vi "Test Analog Channel.vi"(8 "error in (no error)":errorcluster, 9 "Channel (0)":u32, 10 "Test Label":string, 11 "CT Common Tests in":refnum<class "CT Common Tests.lvclass">) -> (0 "error out":errorcluster, 1 "Result":string, 2 "Passed":bool, 3 "CT Common Tests out":refnum<class "CT Common Tests.lvclass">)   [LabVIEW 2015, in "CT Common Tests.lvclass"]
uses:
  CT Common Tests.lvclass
  Classes/Instruments/MIO Device/MIO Device/Class/typedefs/Read Type -- Enum.ctl
  Classes/Instruments/MIO Device/MIO Device/Class/typedefs/Channel Type -- Enum.ctl
  Classes/Instruments/MIO Device/MIO Device/Class/MIO Device.lvclass
  Classes/Application/Class/Application.lvclass
  Classes/Test Recipe/Class/Test Recipe.lvclass
  Test Class/Test Class.lvclass
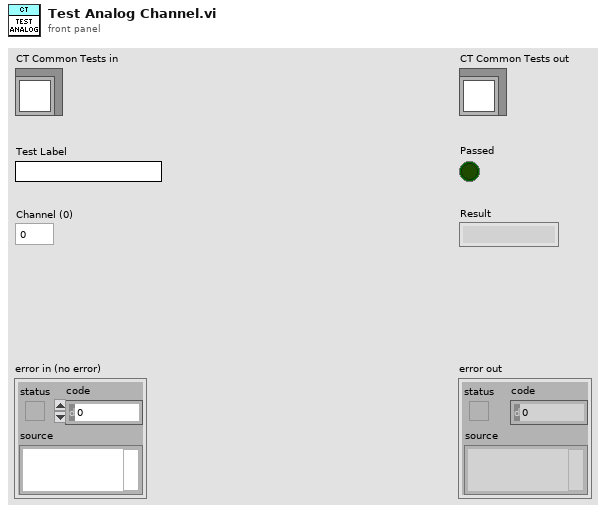
[diagram p1: front panel]
types:
  T1 = typedef "MIO Device.lvlib/MIO Device.lvclass/Channel Type -- Enum.ctl" = enum16{"Analog Input", "Analog Output", "Digital Input", "Digital Output"}
  T2 = typedef "MIO Device.lvlib/MIO Device.lvclass/Read Type -- Enum.ctl" = enum16{"Get All", "Get Latest", "Get Average"}
  T3 = typedef "Application.lvlib/App Properties.lvclass/Class Properties -- Cluster.ctl" = cluster{"UUT Info":T4[], "Test Information":refnum<vi>, "Test Complete Event":refnum<user-event>, "Shop Floor System":refnum<class "Shop Floor System.lvclass">, "Gold Board":refnum<class "Golden Board.lvclass">, "Test Recipe":refnum<class "Test Recipe.lvclass">, "Instruments":refnum<class "Instrument.lvclass">[], "Mode":T5, "Test Results":cluster{"Pass":bool[], "Fail Codes":string[]}, "Station Config":refnum<class "Station Config.lvclass">}
  T4 = typedef "Application.lvlib/App Properties.lvclass/UUT Reference -- Cluster.ctl" = cluster{"Serial Number Reference":refnum<vi>, "Status Message Reference":refnum<vi>}
  T5 = typedef "Application.lvlib/Application.lvclass/Op Mode -- Enum.ctl" = u16
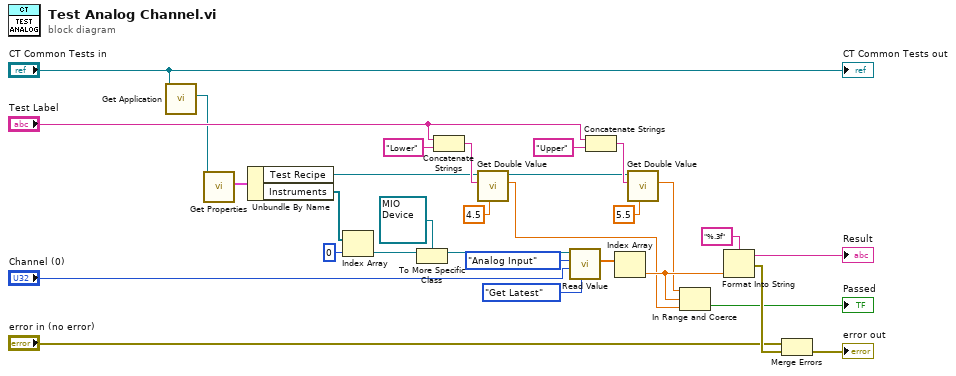
[diagram p0: block diagram]
diagram:
  n1 = call "Get Application.vi"("Test Class in"="CT Common Tests in") -> ("Application.lvlib:Application.lvclass"=w4:refnum<class "Application.lvclass">)  [unwired: 9 in, 1 out]
  n2 = call "Get Properties.vi"("Acrobat Template in"=w4) -> ("Class Properties"=w8:T3)  [unwired: 8 in, 2 out]
  n3 = Unbundle By Name(w8) -> ("Test Recipe"=w12:refnum<class "Test Recipe.lvclass">, "Instruments"=w7:refnum<class "Instrument.lvclass">[])
  n4 = Index Array(array=w7, index=0) -> (element=w5:refnum<class "Instrument.lvclass">)
  n5 = To More Specific Class(target class=refnum<class "MIO Device.lvclass"> refnum ("MIO Device.lvlib:MIO Device.lvclass"), reference=w5) -> (specific class reference=w9:refnum<class "MIO Device.lvclass">)  [unwired: 1 in, 1 out]
  n6 = Concatenate Strings("Test Label", "Lower" ("Name")) -> (w21:string)
  n7 = call "Get Double Value.vi"("Default Value"=4.5, "Name"=w21, "Test Recipe in"=w12) -> ("Value"=w18:dbl, "Test Recipe out"=w13:refnum<class "Test Recipe.lvclass">)  [unwired: 6 in, 1 out]
  n8 = call-dynamic "Read Value.vi"("Read Function (Get All)"=Read_Type_--_Enum."Get Latest", "Channel (0)"="Channel (0)", "Channel Type"=Channel_Type_--_Enum."Analog Input", "MIO Device in"=w9) -> ("First Channel"=w16:dbl[])  [unwired: 4 in, 3 out]
  n9 = Concatenate Strings("Test Label", "Upper" ("Name")) -> (w23:string)
  n10 = Index Array(array=w16) -> (element=w19:dbl)  [unwired: 1 in]
  n11 = call "Get Double Value.vi"("Default Value"=5.5, "Name"=w23, "Test Recipe in"=w13) -> ("Value"=w17:dbl)  [unwired: 6 in, 2 out]
  n12 = In Range and Coerce(upper limit=w17, x=w19, lower limit=w18) -> (In Range?=→"Passed":bool)  [unwired: 1 out]
  n13 = Format Into String(format string="%.3f", w19) -> (resulting string=→"Result":string, error out=w30:errorcluster)  [unwired: 2 in]
  n14 = Merge Errors("error in (no error)", w30) -> (→"error out":errorcluster)
  "CT Common Tests out" <- "CT Common Tests in"
